vi "load_bubble.vi"(8 "error in (no error)":errorcluster, 11 "HTS PORT":refnum<visa-resource-name>) -> (0 "error out":errorcluster, 3 "HTS PORT OUT":refnum<visa-resource-name>)   [LabVIEW 2013]
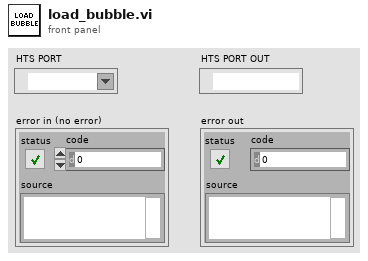
[diagram p1: front panel]
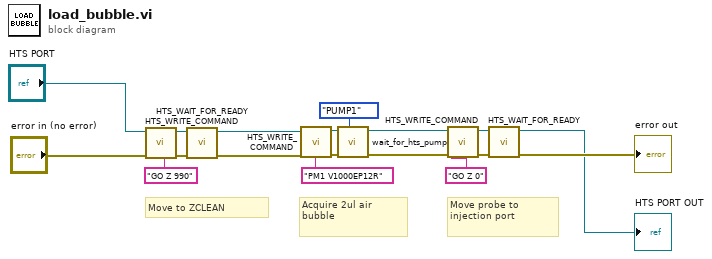
[diagram p0: block diagram]
diagram:
  # "Move probe to \ninjection port"
  # "Acquire 2ul air\nbubble"
  # "Move to ZCLEAN"
  n1 = call "HTS_WRITE_COMMAND.vi"("Error IN"="error in (no error)", "Command"="GO Z 990", "HTS PORT IN"="HTS PORT") -> ("Error OUT"=w4:errorcluster, "HTS PORT OUT"=w5:refnum<visa-resource-name>)  [unwired: 6 in, 1 out]
  n2 = call "HTS_WAIT_FOR_READY.vi"("Error IN"=w4, "VISA resource IN"=w5) -> ("Error OUT"=w7:errorcluster, "VISA resource OUT"=w6:refnum<visa-resource-name>)  [unwired: 6 in, 2 out]
  n3 = call "HTS_WRITE_COMMAND.vi"("Error IN"=w7, "Command"="PM1 V1000EP12R", "HTS PORT IN"=w6) -> ("Error OUT"=w10:errorcluster, "HTS PORT OUT"=w9:refnum<visa-resource-name>)  [unwired: 6 in, 1 out]
  n4 = call "wait_for_hts_pump.vi"("error in (no error)"=w10, "PUMP"=enum16{"PUMP2", "PUMP1"}."PUMP1", "HTS PORT IN"=w9) -> ("error out"=w16:errorcluster, "HTS PORT OUT"=w15:refnum<visa-resource-name>)  [unwired: 7 in]
  n5 = call "HTS_WRITE_COMMAND.vi"("Error IN"=w16, "Command"="GO Z 0", "HTS PORT IN"=w15) -> ("Error OUT"=w13:errorcluster, "HTS PORT OUT"=w14:refnum<visa-resource-name>)  [unwired: 6 in, 1 out]
  n6 = call "HTS_WAIT_FOR_READY.vi"("Error IN"=w13, "VISA resource IN"=w14) -> ("Error OUT"=→"error out":errorcluster, "VISA resource OUT"=→"HTS PORT OUT":refnum<visa-resource-name>)  [unwired: 6 in, 2 out]
